vi "MainVI_IRVision.vi"() -> ()   [LabVIEW 2013]
uses:
  StateEnum.ctl
  StateImageQueue.ctl
  Parameter.ctl
  <vilib>/picture/picture.llb/imagedata.ctl
  <vilib>/Analysis/baseanly.llb/Mean (DBL).vi
  <vilib>/Analysis/NI_AALBase.lvlib
panel:
  out "error out 2":errorcluster caption="error out"
  out "error out":errorcluster
  in  "UPDATE - Button":bool
  out "IRImage Width":i32
  out "IRImage Height":i32
  in  "Camera":u32(ring) items=["t890-2(2131919)"=2131919]
  out "MEASUREMENT RANGES":u32
  out "Min. Value":sgl format="%#_2f"
  out "Max. Value":sgl format="%#_2f"
  out "Mean":dbl caption="Mittelwert" format="%0.2f"
  in  "PaletteType":u8(ring) items=["Iron", "Rainbow", "BlueRed", "Testo", "Sepia", "Dewpoint", "RainbowHC"]
  out "IsStreaming":bool
  out "CONNECTED":bool caption="l"
  in  "STOP - Button":bool
  in  "SAVE - Button":bool
  in  "CONNECT - Button":bool
  in  "STREAM - Button":bool
  in  "EXIT - Button":bool
  in  "ATMOSPHERECORRECTION":bool
  in  "AMBIENTTEMPERATURE":sgl
  in  "HUMIDITY":sgl
  in  "MEASUREMENT RANGE":u32
  in  "REFLECTEDTEMPERATURE":sgl
  in  "EMISSIVITY":sgl=0.3 format="%.2f"
  out "IR Image":picture
  # "Testo 885, 890"
  # "CONNECTION"
  # "STREAM"
  # "PARAMETER"
  # "IR IMAGE"
  # "Measurement Ranges"
  # "Palette Type"
  # "Measurement Range"
  # "Height"
  # "Humidity"
  # "Width"
  # "Ambient Temperature"
  # "Min. Value"
  # "Emissivity"
  # "Max. Value"
  # "Reflected Temperature"
  # "Mean Value"
  # "Atmosphere Correction"
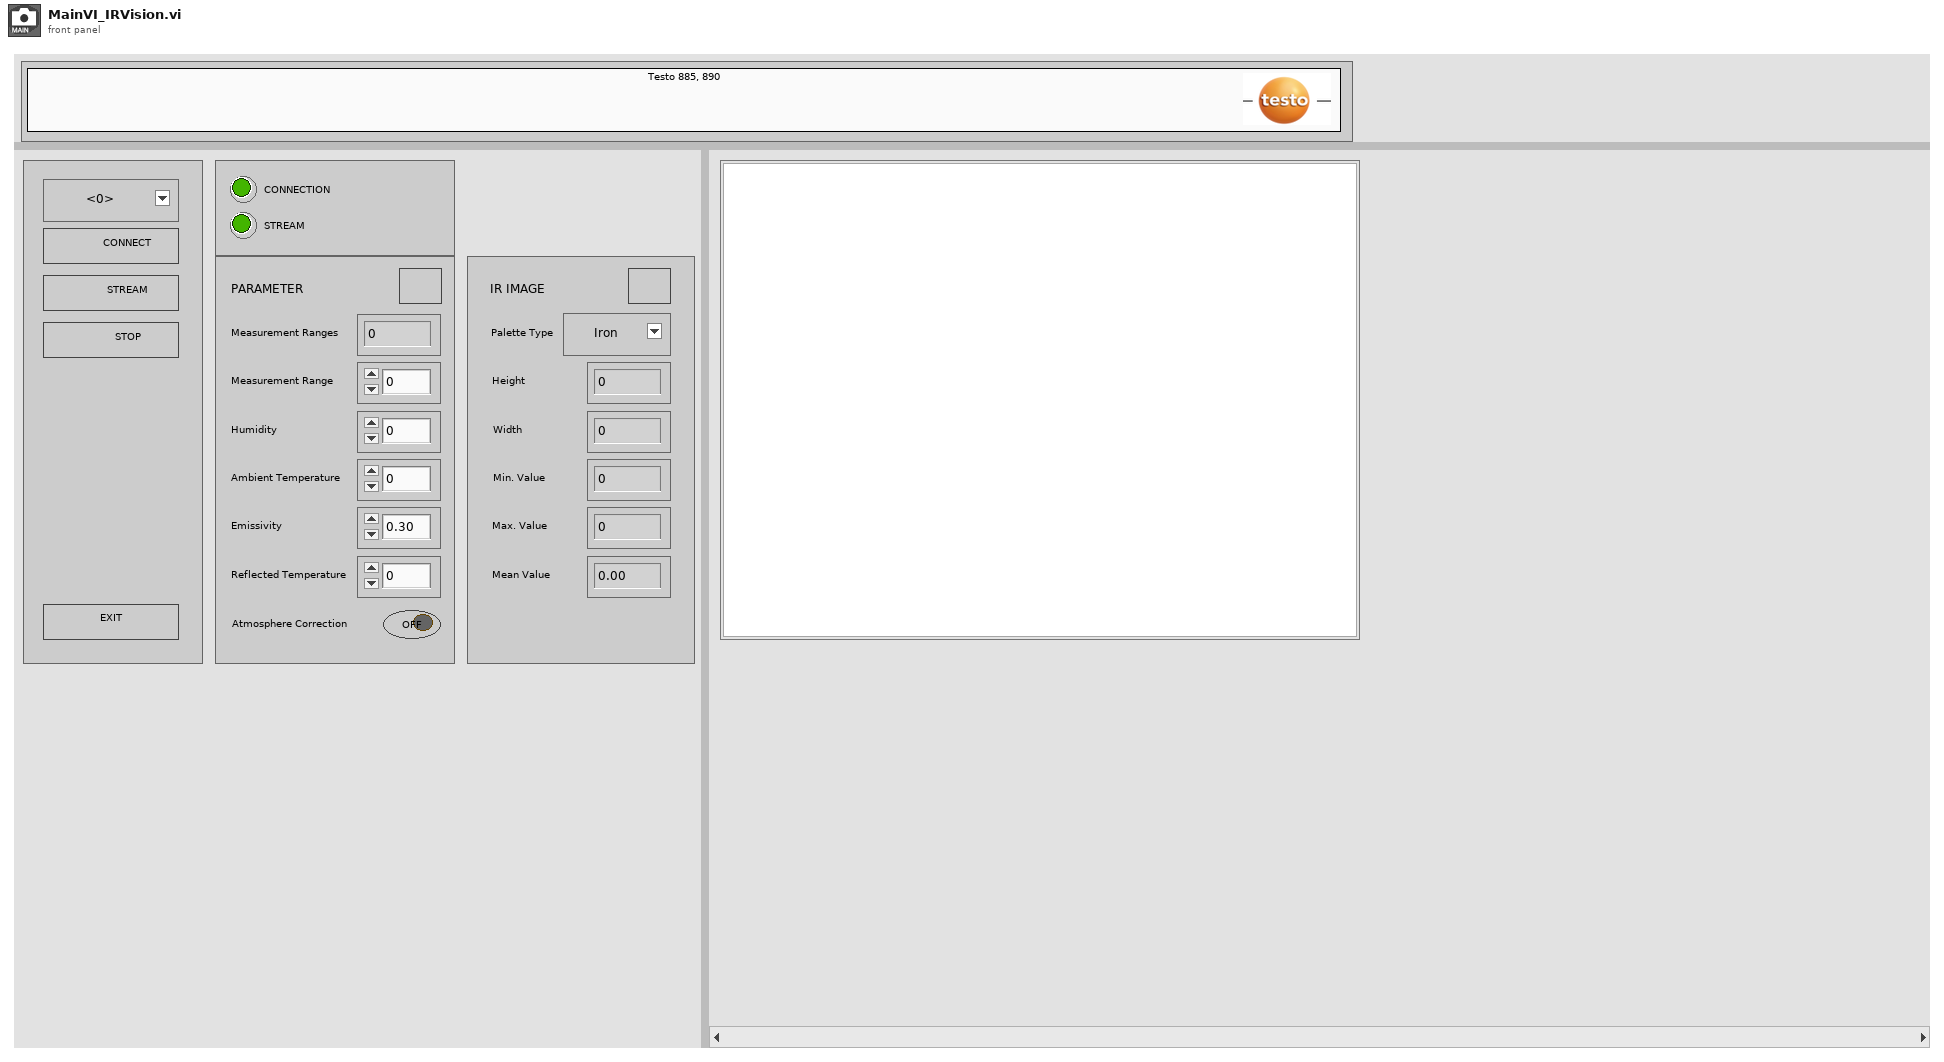
[diagram p1: front panel]
types:
  T1 = typedef "StateImageQueue.ctl" = enum16{"INITIALIZE", "GET IMAGE", "IDLE", "GET STREAM", "EXIT", ""}
  T2 = typedef "StateEnum.ctl" = enum16{"INITIALIZE", "CONNECT", "STREAM", "STOPSTREAM", "GETIMAGES", "SETPARAMTER", "GETPARAMETER", "SAVEIMAGE", "EXIT"}
  T3 = cluster{"IR QUEUE":refnum<queue>, "VIS QUEUE":refnum<queue>}
  T4 = typedef "Parameter.ctl" = enum16{"EMISSIVITY", "ATMOSPHERECORRECTION", "HUMIDITY", "REFLECTEDTEMPERATURE", "AMBIENTTEMPERATURE", "MEASUREMENTRANGE"}
  T5 = typedef "imagedata.ctl" = cluster{"image type":i32, "image depth":i32, "image":u8[], "mask":u8[], "colors":u32[], "Rectangle":cluster{"left":i16, "top":i16, "right":i16, "bottom":i16}}
  T6 = cluster{"left":i16, "top":i16, "right":i16, "bottom":i16}
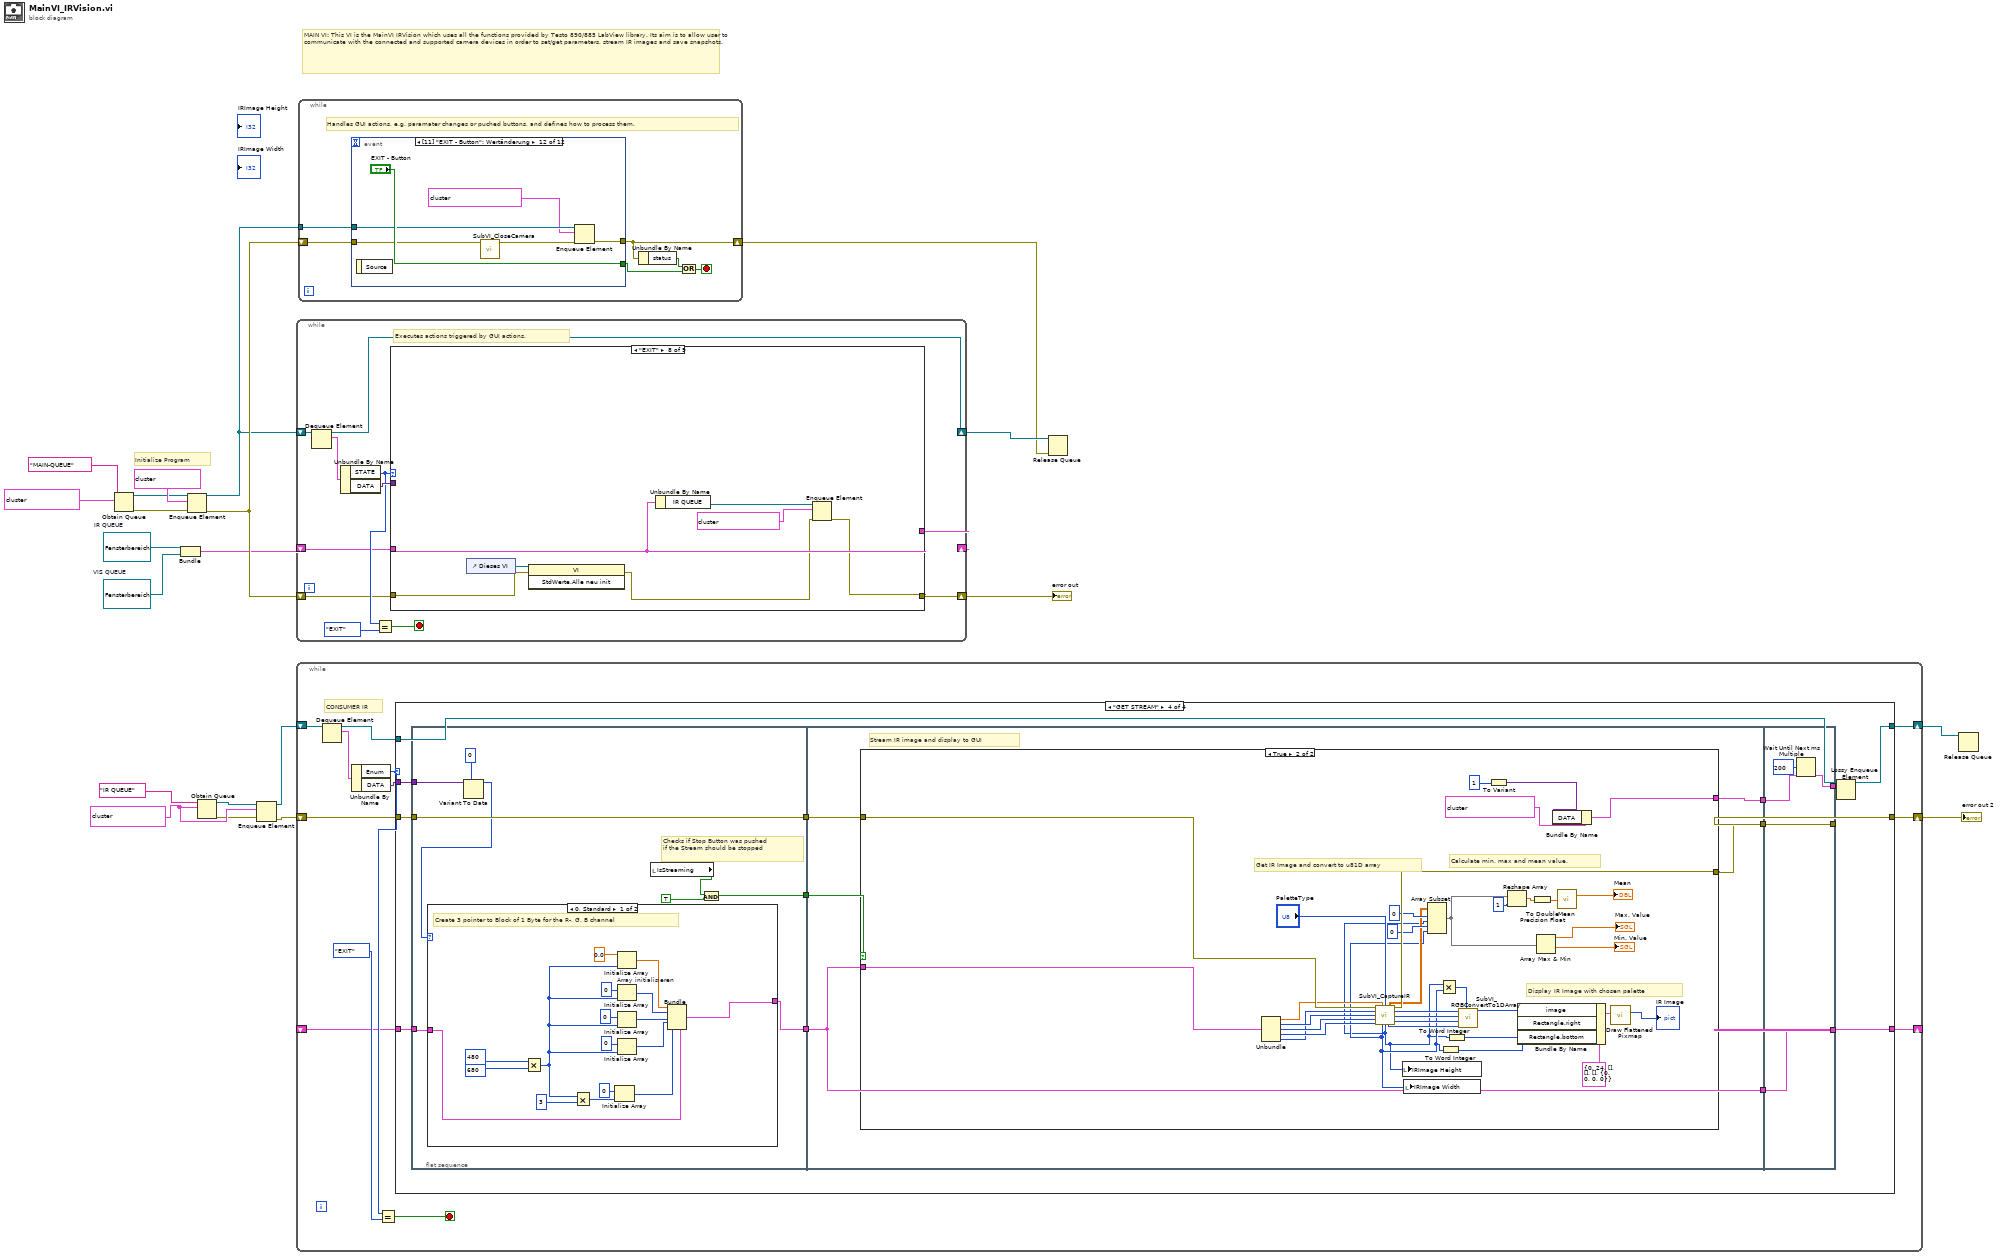
[diagram p0: block diagram]
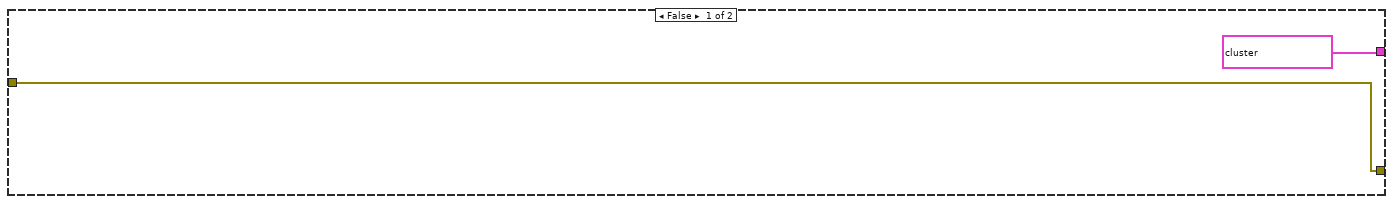
[diagram p6: hidden frame]
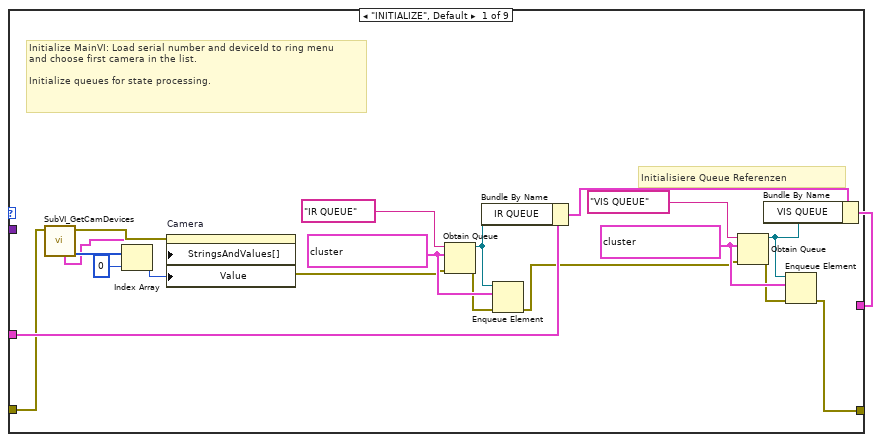
[diagram p7: hidden frame]
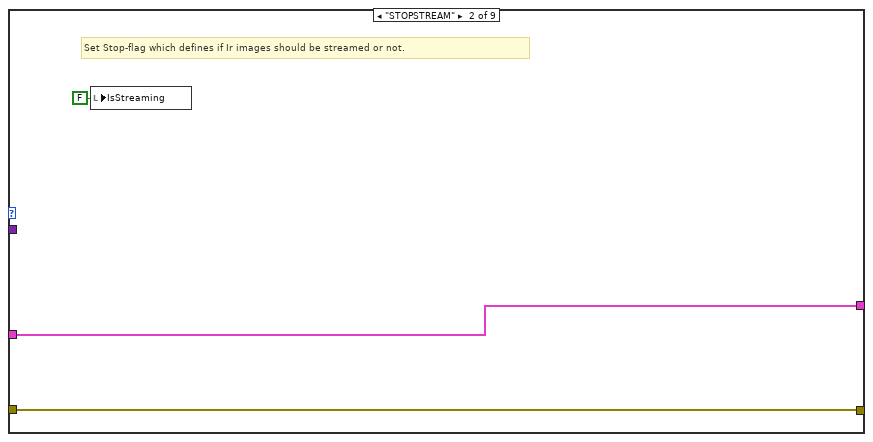
[diagram p8: hidden frame]
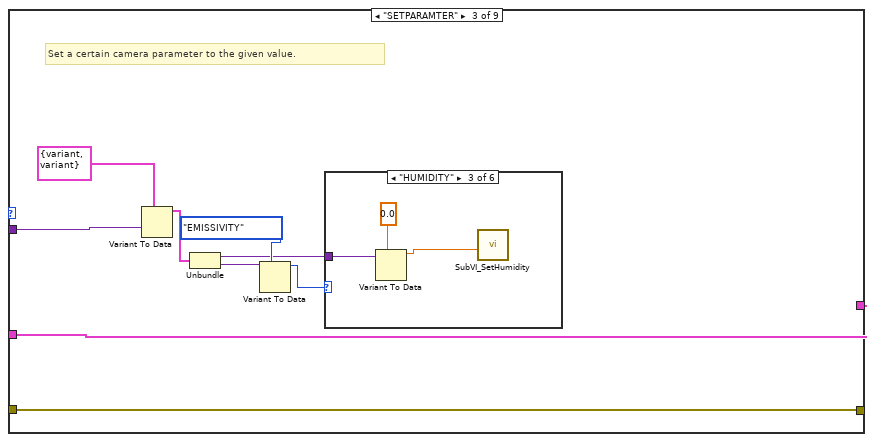
[diagram p9: hidden frame]
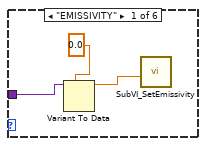
[diagram p10: hidden frame]
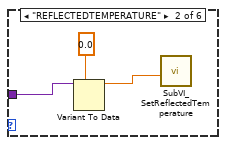
[diagram p11: hidden frame]
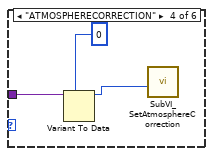
[diagram p12: hidden frame]
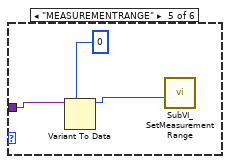
[diagram p13: hidden frame]
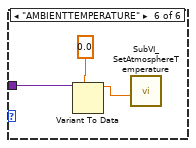
[diagram p14: hidden frame]
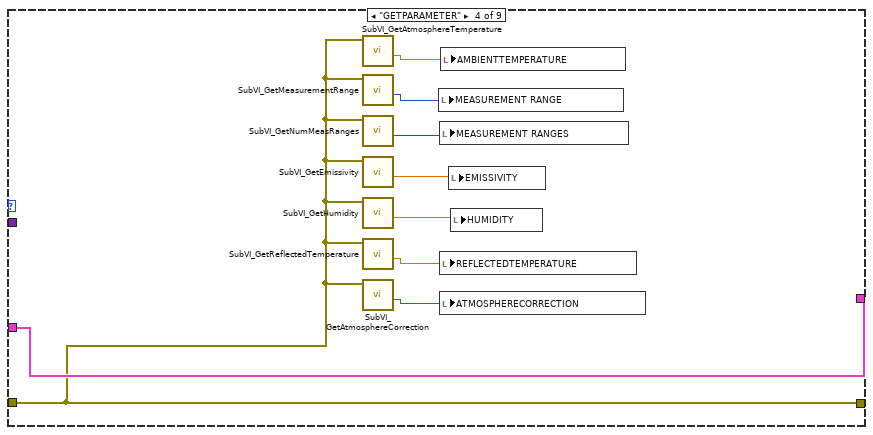
[diagram p15: hidden frame]
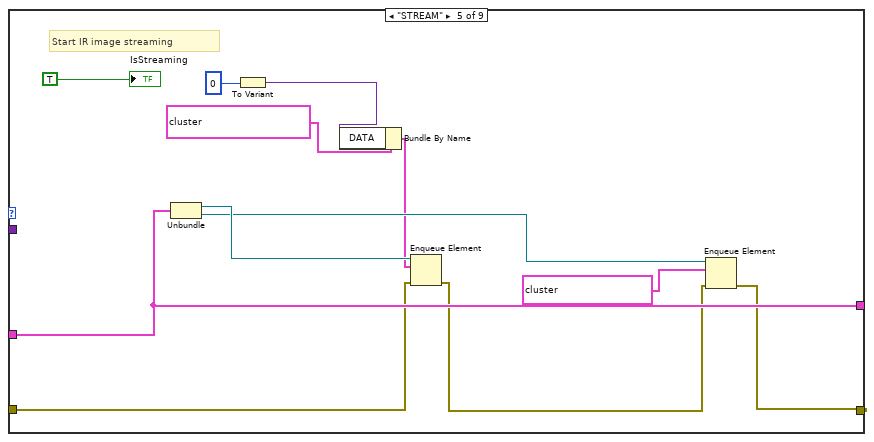
[diagram p16: hidden frame]
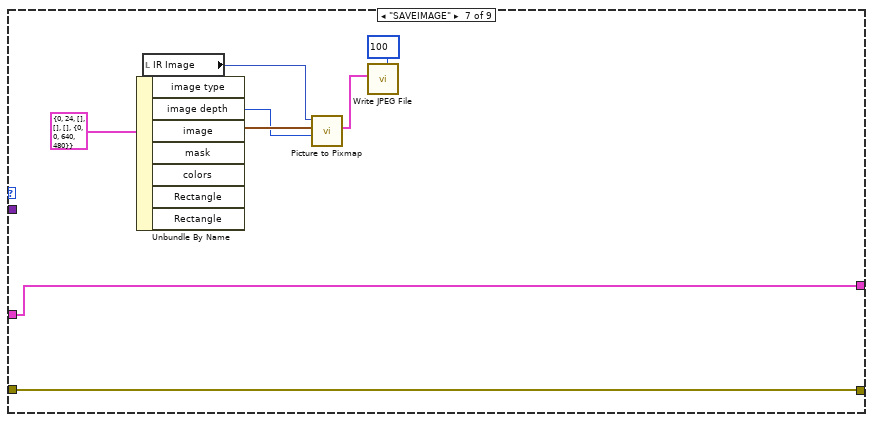
[diagram p18: hidden frame]
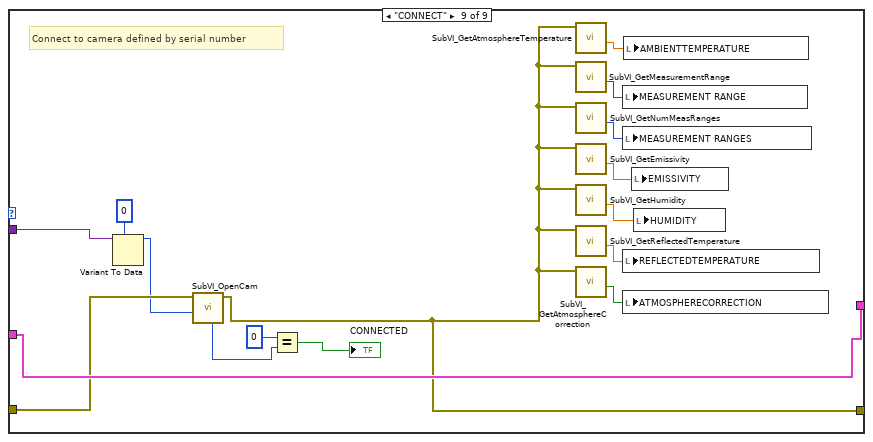
[diagram p19: hidden frame]
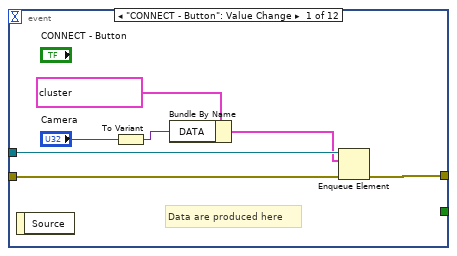
[diagram p20: hidden frame]
diagram:
  w3 = refnum<queue> refnum  # VIS QUEUE
  w7 = refnum<queue> refnum  # IR QUEUE
  w13 = cluster{"DATA":variant, "Enum":T1} {"DATA"=variant, "Enum"=enum."INITIALIZE"}
  # "Initialize Program"
  # "MAIN VI: This VI is the MainVI IRVision which uses all the functions provided by Testo 890/885 LabView library. Its aim is to allow user to communicate with the connected and supported camera devices in order to set/get parameters, stream IR images and save snapshots."
  n1 = Obtain Queue(name (unnamed)="MAIN-QUEUE" ("Name (unbenannt)"), element data type=cluster{"DATA":variant, "STATE":T2} {"DATA"=variant, "STATE"=enum."INITIALIZE"}) -> (queue out=w18:refnum<queue>, error out=w17:errorcluster)  [unwired: 3 in, 1 out]
  n2 = Bundle("IR QUEUE"=w7, "VIS QUEUE"=w3) -> (w6:T3)  [unwired: 1 in]
  n3 = Enqueue Element(queue=w18, element=cluster{"DATA":variant, "STATE":T2} {"DATA"=variant, "STATE"=enum."INITIALIZE"} ("Element"), error in (no error)=w17) -> (queue out=w11:refnum<queue>, error out=w16:errorcluster)  [unwired: 1 in, 1 out]
  n4 = Obtain Queue(name (unnamed)="IR QUEUE" ("Name (unbenannt)"), element data type=w13) -> (queue out=w14:refnum<queue>, error out=w12:errorcluster)  [unwired: 3 in, 1 out]
  n5 = Enqueue Element(queue=w14, element=w13, error in (no error)=w12) -> (queue out=w5:refnum<queue>, error out=w4:errorcluster)  [unwired: 1 in, 1 out]
  n6 = while {
    shift-right: [w24] -> w1
    shift-left: w16 -> [w27]
    shift-right: [w22] -> w10
    shift-left: w11 -> [w32]
    shift-right: [w25] -> _
    shift-left: w6 -> [w26]
    stop <- w23 stop-if-true
    # "Executes actions triggered by GUI actions."
    n7 = Dequeue Element(queue=w32) -> (queue out=w22:refnum<queue>, element=w31:cluster{"DATA":variant, "STATE":T2})  [unwired: 2 in, 2 out]
    n8 = Unbundle By Name(w31) -> ("STATE"=w29:T2, "DATA"=w30:variant)
    n9 = Equal?(x=w29, y=StateEnum."EXIT") -> (x = y?=w23:bool)
    n10 = case shown="\"EXIT\"" w29 {
      tunnel: w30 -> [_ _ w64 _ _ _ _ _ w135]
      tunnel: w27 -> [w34 w54 w56 w90 w101 w104 w106 w116 w133]
      tunnel: [w38 w54 w56 w90 w96 w104 w106 w114 w132] -> w24
      tunnel: w26 -> [w47 w55 w63 w91 w103 w105 w107 w118 w134]
      tunnel: [w35 w55 w63 w91 w103 w105 w107 w118 w134] -> w25
      frame "INITIALIZE", Default {
        w41 = cluster{"DATA":variant, "Enum":T1} {"DATA"=variant, "Enum"=enum."INITIALIZE"}
        w46 = cluster{"DATA":variant, "Enum":T1} {"DATA"=variant, "Enum"=enum."INITIALIZE"}
        # "Initialisiere Queue Referenzen"
        # "Initialize MainVI: Load serial number and deviceId to ring menu\nand choose first camera in the list.\n\nInitialize queues for state processing."
        n11 = call "SubVI_GetCamDevices.vi"("ErrorIn"=w34) -> ("au32CameraSerials"=w51:u32[], "ErrorOut"=w49:errorcluster, "strCameraDeviceType"=w33:cluster{string, "Output":u32}[])  [unwired: 6 in, 2 out]
        n12 = Index Array(array=w51, index=0 ("Index")) -> (element=w52:u32)
        n13 = property on="Camera" class="Ring (strikt)"(error in=w49, "StringsAndValues[]"=w33, "Value"=w52) -> (error out=w43:errorcluster)  [unwired: 1 in, 1 out]
        n14 = Obtain Queue ("Queue anfordern")(name (unnamed)="IR QUEUE" ("Name (unbenannt)"), element data type=w46, error in (no error)=w43) -> (queue out=w45:refnum<queue>, error out=w44:errorcluster)  [unwired: 2 in, 1 out]
        n15 = Bundle By Name(cluster=w47, "IR QUEUE"=w45) -> (w36:T3)
        n16 = Enqueue Element(queue=w45, element=w46, error in (no error)=w44) -> (error out=w39:errorcluster)  [unwired: 1 in, 2 out]
        n17 = Obtain Queue ("Queue anfordern")(name (unnamed)="VIS QUEUE" ("Name (unbenannt)"), element data type=w41, error in (no error)=w39) -> (queue out=w37:refnum<queue>, error out=w40:errorcluster)  [unwired: 2 in, 1 out]
        n18 = Bundle By Name(cluster=w36, "VIS QUEUE"=w37) -> (w35:T3)
        n19 = Enqueue Element(queue=w37, element=w41, error in (no error)=w40) -> (error out=w38:errorcluster)  [unwired: 1 in, 2 out]
      }
      frame "STOPSTREAM" {
        # "Set Stop-flag which defines if Ir images should be streamed or not."
        n20 = local write "IsStreaming"(FALSE) -> ()
      }
      frame "SETPARAMTER" {
        # "Set a certain camera parameter to the given value."
        n21 = Variant To Data(type=cluster{variant, variant} {variant, variant}, Variant=w64) -> (data=w61:cluster{variant, variant})  [unwired: 1 in, 1 out]
        n22 = Unbundle(w61) -> (w57:variant, w58:variant)
        n23 = Variant To Data(type=Parameter."EMISSIVITY" ("Enum"), Variant=w58) -> (data=w59:T4)  [unwired: 1 in, 1 out]
        n24 = case shown="\"HUMIDITY\"" w59 {
          tunnel: w57 -> [w67 w69 w72 w76 w78 w81]
          frame "EMISSIVITY" {
            n25 = Variant To Data(type=sgl 0.0, Variant=w67) -> (data=w65:sgl)  [unwired: 1 in, 1 out]
            n26 = call "SubVI_SetEmissivity.vi"("fEmissivity"=w65) -> ()  [unwired: 9 in, 2 out]
          }
          frame "REFLECTEDTEMPERATURE" {
            n27 = Variant To Data(type=sgl 0.0, Variant=w69) -> (data=w68:sgl)  [unwired: 1 in, 1 out]
            n28 = call "SubVI_SetReflectedTemperature.vi"("fReflectedTemp"=w68) -> ()  [unwired: 9 in, 2 out]
          }
          frame "HUMIDITY" {
            n29 = Variant To Data(type=sgl 0.0, Variant=w72) -> (data=w71:sgl)  [unwired: 1 in, 1 out]
            n30 = call "SubVI_SetHumidity.vi"("fHumidity"=w71) -> ()  [unwired: 9 in, 2 out]
          }
          frame "ATMOSPHERECORRECTION" {
            n31 = Variant To Data(type=u8 0, Variant=w76) -> (data=w74:u8)  [unwired: 1 in, 1 out]
            n32 = call "SubVI_SetAtmosphereCorrection.vi"("u8AtmosCorrEnable"=w74) -> ()  [unwired: 9 in, 2 out]
          }
          frame "MEASUREMENTRANGE" {
            n33 = Variant To Data(type=u32 0, Variant=w78) -> (data=w77:u32)  [unwired: 1 in, 1 out]
            n34 = call "SubVI_SetMeasurementRange.vi"("u32MeasurementRange"=w77) -> ()  [unwired: 9 in, 2 out]
          }
          frame "AMBIENTTEMPERATURE" {
            n35 = Variant To Data(type=sgl 0.0, Variant=w81) -> (data=w80:sgl)  [unwired: 1 in, 1 out]
            n36 = call "SubVI_SetAtmosphereTemperature.vi"("fAtmosTemp"=w80) -> ()  [unwired: 9 in, 2 out]
          }
        }
      }
      frame "GETPARAMETER" {
        n37 = call "SubVI_GetAtmosphereTemperature.vi"("ErrorIn"=w90) -> ("fAtmosTemp"=w89:sgl)  [unwired: 8 in, 2 out]
        n38 = call "SubVI_GetMeasurementRange.vi"("ErrorIn"=w90) -> ("u32MeasRangeIndex"=w88:u32)  [unwired: 8 in, 2 out]
        n39 = call "SubVI_GetNumMeasRanges.vi"("ErrorIn"=w90) -> ("u32NumMeasRanges"=w87:u32)  [unwired: 8 in, 2 out]
        n40 = call "SubVI_GetEmissivity.vi"("ErrorIn"=w90) -> ("fEmissivity"=w86:sgl)  [unwired: 8 in, 2 out]
        n41 = call "SubVI_GetHumidity.vi"("ErrorIn"=w90) -> ("fHumidity"=w85:sgl)  [unwired: 8 in, 2 out]
        n42 = call "SubVI_GetReflectedTemperature.vi"("ErrorIn"=w90) -> ("fReflectedTemp"=w84:sgl)  [unwired: 8 in, 2 out]
        n43 = call "SubVI_GetAtmosphereCorrection.vi"("ErrorIn"=w90) -> ("bAtmosCorrEnable"=w83:bool)  [unwired: 8 in, 2 out]
        n44 = local write "MEASUREMENT RANGE"(w88) -> ()
        n45 = local write "MEASUREMENT RANGES"(w87) -> ()
        n46 = local write "REFLECTEDTEMPERATURE"(w84) -> ()
        n47 = local write "ATMOSPHERECORRECTION"(w83) -> ()
        n48 = local write "AMBIENTTEMPERATURE"(w89) -> ()
        n49 = local write "EMISSIVITY"(w86) -> ()
        n50 = local write "HUMIDITY"(w85) -> ()
      }
      frame "STREAM" {
        # "Start IR image streaming"
        n51 = Unbundle(w103) -> ("IR QUEUE"=w102:refnum<queue>, "VIS QUEUE"=w98:refnum<queue>)
        n52 = To Variant(anything=u8 0) -> (Variant=w95:variant)
        n53 = Bundle By Name(cluster=cluster{"DATA":variant, "Enum":T1} {"DATA"=variant, "Enum"=enum."GET STREAM"}, "DATA"=w95) -> (w92:cluster{"DATA":variant, "Enum":T1})
        n54 = Enqueue Element(queue=w102, element=w92, error in (no error)=w101) -> (error out=w97:errorcluster)  [unwired: 1 in, 2 out]
        n55 = Enqueue Element(queue=w98, element=cluster{"DATA":variant, "Enum":T1} {"DATA"=variant, "Enum"=enum."GET STREAM"}, error in (no error)=w97) -> (error out=w96:errorcluster)  [unwired: 1 in, 2 out]
        "IsStreaming" <- TRUE
      }
      frame "GETIMAGES" {
      }
      frame "SAVEIMAGE" {
        n56 = Unbundle By Name(T5 {"image type"=0, "image depth"=24, "image"=[], "mask"=[], "colors"=[], "Rectangle"={"left"=0, "top"=0, "right"=640, "bottom"=480}} ("image data")) -> ("image depth"=w110:i32, "Rectangle"=w112:T6)  [unwired: 5 out]
        n57 = local read "IR Image"() -> (w111:picture)
        n58 = call <vilib>:"Picture to Pixmap.vi"("depth"=w110, "rect"=w112, "picture"=w111) -> ("image data"=w109:T5)  [unwired: 7 in, 1 out]
        n59 = call <vilib>:"Write JPEG File.vi"("quality (80)"=100, "image data"=w109) -> ()  [unwired: 8 in, 2 out]
      }
      frame "EXIT" {
        n60 = control-ref of="Dieses VI"() -> (w117:refnum<vi>)
        n61 = invoke class="VI" method="StdWerte.Alle neu init"(reference=w117, error in=w116) -> (error out=w115:errorcluster)  [unwired: 1 in, 2 out]
        n62 = Unbundle By Name(w118) -> ("IR QUEUE"=w119:refnum<queue>)
        n63 = Enqueue Element(queue=w119, element=cluster{"DATA":variant, "Enum":T1} {"DATA"=variant, "Enum"=enum."EXIT"}, error in (no error)=w115) -> (error out=w114:errorcluster)  [unwired: 1 in, 2 out]
      }
      frame "CONNECT" {
        # "Connect to camera defined by serial number"
        n64 = Variant To Data(type=u32 0 ("Typ"), Variant=w135) -> (data=w131:u32)  [unwired: 1 in, 1 out]
        n65 = call "SubVI_OpenCam.vi"("u32SerialNumber"=w131, "ErrorIn"=w133) -> ("ErrorOut"=w132:errorcluster, "u8Status"=w123:u8)  [unwired: 8 in]
        n66 = Equal?(x=u8 0, y=w123) -> (x = y?=→"CONNECTED":bool)
        n67 = call "SubVI_GetAtmosphereTemperature.vi"("ErrorIn"=w132) -> ("fAtmosTemp"=w124:sgl)  [unwired: 8 in, 2 out]
        n68 = call "SubVI_GetMeasurementRange.vi"("ErrorIn"=w132) -> ("u32MeasRangeIndex"=w125:u32)  [unwired: 8 in, 2 out]
        n69 = call "SubVI_GetNumMeasRanges.vi"("ErrorIn"=w132) -> ("u32NumMeasRanges"=w126:u32)  [unwired: 8 in, 2 out]
        n70 = call "SubVI_GetEmissivity.vi"("ErrorIn"=w132) -> ("fEmissivity"=w127:sgl)  [unwired: 8 in, 2 out]
        n71 = call "SubVI_GetHumidity.vi"("ErrorIn"=w132) -> ("fHumidity"=w128:sgl)  [unwired: 8 in, 2 out]
        n72 = call "SubVI_GetReflectedTemperature.vi"("ErrorIn"=w132) -> ("fReflectedTemp"=w129:sgl)  [unwired: 8 in, 2 out]
        n73 = call "SubVI_GetAtmosphereCorrection.vi"("ErrorIn"=w132) -> ("bAtmosCorrEnable"=w130:bool)  [unwired: 8 in, 2 out]
        n74 = local write "MEASUREMENT RANGE"(w125) -> ()
        n75 = local write "MEASUREMENT RANGES"(w126) -> ()
        n76 = local write "REFLECTEDTEMPERATURE"(w129) -> ()
        n77 = local write "ATMOSPHERECORRECTION"(w130) -> ()
        n78 = local write "AMBIENTTEMPERATURE"(w124) -> ()
        n79 = local write "EMISSIVITY"(w127) -> ()
        n80 = local write "HUMIDITY"(w128) -> ()
      }
    }
  }
  "error out" <- w1
  n81 = while {
    shift-right: [w137] -> w8
    shift-left: w5 -> [w144]
    shift-right: [w142] -> w2
    shift-left: w4 -> [w141]
    shift-right: [w139] -> _
    shift-left: _ -> [w140]
    stop <- w146 stop-if-true
    # "CONSUMER IR"
    n82 = Dequeue Element(queue=w144) -> (queue out=w138:refnum<queue>, element=w148:cluster{"DATA":variant, "Enum":T1})  [unwired: 2 in, 2 out]
    n83 = Unbundle By Name(w148) -> ("Enum"=w145:T1, "DATA"=w147:variant)
    n84 = Equal?(x=w145, y=StateImageQueue."EXIT" ("Enum 2")) -> (x = y?=w146:bool)
    n85 = case shown="\"GET STREAM\"" w145 {
      tunnel: w147 -> [_ _ _ w158]
      tunnel: [w151 w154 w157 w168] -> w142
      tunnel: w141 -> [w151 w154 w157 w170]
      tunnel: w140 -> [w150 w152 w156 w167]
      tunnel: [w150 w152 w156 w166] -> w139
      tunnel: w138 -> [w149 w153 w155 w162]
      tunnel: [w149 w153 w155 w163] -> w137
      frame "INITIALIZE", Default {
        # "Initialize ring menu with serial numbers\nand choose first camera in the list"
      }
      frame "IDLE" {
      }
      frame "GET IMAGE" {
      }
      frame "GET STREAM" {
        n86 = flat-sequence {
          tunnel: w167 -> [w172]
          tunnel: w170 -> [w180]
          tunnel: [w180] -> w161
          tunnel: [w173] -> w160
          tunnel: [w177] -> w159
          tunnel: w158 -> [w175]
          tunnel: [w201] -> w171
          tunnel: [w202] -> w169
          tunnel: [w200] -> w165
          tunnel: w161 -> [w203]
          tunnel: w160 -> [w200]
          tunnel: w159 -> [w199]
          tunnel: w171 -> [w241]
          tunnel: w169 -> [w243]
          tunnel: [w243] -> w168
          tunnel: [w244] -> w166
          tunnel: w165 -> [w244]
          tunnel: [w241] -> w164
          frame #0 {
            # "Checks if Stop Button was pushed\nif the Stream should be stopped"
            n87 = Variant To Data(type=u8 0 ("Typ"), Variant=w175) -> (data=w174:u8)  [unwired: 1 in, 1 out]
            n88 = case shown="0, Standard" w174 {
              tunnel: [w187 w198] -> w173
              tunnel: w172 -> [w186 w198]
              frame 0, Default {
                # "Create 3 pointer to Block of 1 Byte for the R-, G, B channel"
                n89 = Multiply(x=480, y=680 ("x")) -> (x*y=w182:i32)
                n90 = Multiply(x=w182, y=3) -> (x*y=w192:i32)
                n91 = Initialize Array(u8 0 ("Element"), w192) -> (w188:u8[])
                n92 = Initialize Array(sgl 0.0 ("Element"), w182) -> (w181:sgl[])
                n93 = Initialize Array "Array initialisieren"(u8 0 ("Element"), w182) -> (w191:u8[])
                n94 = Initialize Array(u8 0 ("Element"), w182) -> (w190:u8[])
                n95 = Initialize Array(u8 0 ("Element"), w182) -> (w189:u8[])
                n96 = Bundle(cluster=w186, w181, w191, w190, w189, w188) -> (w187:cluster{sgl[], u8[], u8[], u8[], u8[]})
              }
              frame 1 {
              }
            }
            n97 = local read "IsStreaming"() -> (w179:bool)
            n98 = And(x=w179, y=TRUE) -> (x .and. y?=w177:bool)
          }
          frame #1 {
            # "Stream IR image and display to GUI"
            n99 = case shown="True" w199 {
              tunnel: w203 -> [w204 w240]
              tunnel: [w204 w239] -> w202
              tunnel: [cluster{"DATA":variant, "Enum":T1} {"DATA"=variant, "Enum"=enum."IDLE"} w216] -> w201
              tunnel: w200 -> [_ w238]
              frame False {
              }
              frame True {
                # "Get IR Image and convert to u81D array"
                # "Calculate min, max and mean value."
                # "Display IR Image with chosen palette"
                n100 = Unbundle(w238) -> (w233:sgl[], w232:u8[], w231:u8[], w230:u8[], w229:u8[])
                n101 = call "SubVI_CaptureIR.vi"("ErrorIn"=w240, "af1DTempMat"=w233, "u8PaletteType"="PaletteType", "au8Channel-B"=w232, "au8Channel-G"=w231, "au8Channel-R"=w230) -> ("af2DTempMat"=w209:sgl[][], "ErrorOut"=w239:errorcluster, "au8Channel-B"=w235:u8[], "au8Channel-G"=w236:u8[], "i32Width"=w207:i32, "i32Height"=w206:i32, "au8Channel-R"=w237:u8[])  [unwired: 2 in, 1 out]
                n102 = local write "IRImage Height"(w206) -> ()
                n103 = local write "IRImage Width"(w207) -> ()
                n104 = Array Subset(array=w209, index (row)=0 ("Index"), length (row)=w206, index (col)=0 ("Index"), length (col)=w207) -> (w208:sgl[][])
                n105 = Multiply(x=w206, y=w207) -> (x*y=w234:i32)
                n106 = To Word Integer(number=w207) -> (16bit integer=w213:i16)
                n107 = To Word Integer(number=w206) -> (16bit integer=w212:i16)
                n108 = call "SubVI_RGBConvertTo1DArray.vi"("i32PixelAmount"=w234, "au8Channel-R"=w237, "au8Channel-G"=w236, "au8Channel-B"=w235, "au8SerializedImage[in]"=w229) -> ("au8SerializedImage[out]"=w226:u8[])  [unwired: 6 in]
                n109 = To Variant(anything=u8 1) -> (Variant=w218:variant)
                n110 = Reshape Array(w208, 1 ("Dimension")) -> (w222:sgl[])
                n111 = Bundle By Name(cluster=T5 {"image type"=0, "image depth"=24, "image"=[], "mask"=[], "colors"=[], "Rectangle"={"left"=0, "top"=0, "right"=0, "bottom"=0}} ("image data"), "image"=w226, "Rectangle.right"=w213, "Rectangle.bottom"=w212) -> (w224:T5)
                n112 = To Double Precision Float(number=w222) -> (double precision float=w223:dbl[])
                n113 = Array Max & Min(array=w208) -> (max value=→"Max. Value":sgl, min value=→"Min. Value":sgl)  [unwired: 2 out]
                n114 = Bundle By Name(cluster=cluster{"DATA":variant, "Enum":T1} {"DATA"=variant, "Enum"=enum."GET STREAM"}, "DATA"=w218) -> (w216:cluster{"DATA":variant, "Enum":T1})
                n115 = call-poly <vilib>:"Mean.vi"("X"=w223) -> ("mean"=→"Mean":dbl)  [unwired: 1 out]
                n116 = call <vilib>:"Draw Flattened Pixmap.vi"("image data"=w224) -> ("new picture"=→"IR Image":picture)  [unwired: 8 in]
              }
            }
          }
          frame #2 {
            n117 = Wait Until Next ms Multiple(millisecond multiple=u32 200 ("ms")) -> ()  [unwired: 1 out]
          }
        }
        n118 = Lossy Enqueue Element(queue=w162, element=w164) -> (queue out=w163:refnum<queue>)  [unwired: 1 in, 3 out]
      }
    }
  }
  "error out 2" <- w2
  n119 = while {
    shift-right: [w245] -> w9
    shift-left: w16 -> [w249]
    tunnel: w11 -> [w250]
    stop <- w248 stop-if-true
    # "Handles GUI actions, e.g. paramater changes or puched buttons, and defines how to process them."
    n120 = event shown="[11] \"EXIT - Button\": Wertänderung" {
      selector: _ -> [_ _ _ _ _ _ _ _ _ _ _ _]
      dyn-events: _ -> [_ _ _ _ _ _ _ _ _ _ _ _]
      timeout: _ -> [_ _ _ _ _ _ _ _ _ _ _ _]
      tunnel: w250 -> [w257 w260 w264 w266 w273 w287 w296 w304 w310 w312 w323 w334]
      tunnel: w249 -> [w256 w261 w263 w267 w272 w286 w295 w303 w309 w313 w322 w331]
      tunnel: [_ _ _ _ _ _ _ _ _ _ _ "EXIT - Button"] -> w246
      tunnel: [w255 w259 w262 w268 w271 w285 w294 w300 w308 w314 w321 w333] -> w245
      event "CONNECT - Button": Value Change {
        # "Data are produced here"
        n121 = event-data() -> ()  [unwired: 1 in, 1 out]
        n122 = To Variant(anything="Camera") -> (Variant=w252:variant)
        n123 = Bundle By Name(cluster=cluster{"DATA":variant, "STATE":T2} {"DATA"=variant, "STATE"=enum."CONNECT"} ("Element"), "DATA"=w252) -> (w251:cluster{"DATA":variant, "STATE":T2})
        n124 = Enqueue Element(queue=w257, element=w251, error in (no error)=w256) -> (error out=w255:errorcluster)  [unwired: 1 in, 2 out]
      }
      event "STREAM - Button": Value Change {
        n125 = event-data() -> ()  [unwired: 1 in, 1 out]
        n126 = Enqueue Element(queue=w260, element=cluster{"DATA":variant, "STATE":T2} {"DATA"=variant, "STATE"=enum."STREAM"} ("Element"), error in (no error)=w261) -> (error out=w259:errorcluster)  [unwired: 1 in, 2 out]
      }
      event "STOP - Button": Value Change {
        n127 = event-data() -> ()  [unwired: 1 in, 1 out]
        n128 = Enqueue Element(queue=w264, element=cluster{"DATA":variant, "STATE":T2} {"DATA"=variant, "STATE"=enum."STOPSTREAM"} ("Element"), error in (no error)=w263) -> (error out=w262:errorcluster)  [unwired: 1 in, 2 out]
      }
      event "UPDATE - Button": Value Change {
        n129 = event-data() -> ()  [unwired: 1 in, 1 out]
        n130 = Enqueue Element(queue=w266, element=cluster{"DATA":variant, "STATE":T2} {"DATA"=variant, "STATE"=enum."GETPARAMETER"} ("Element"), error in (no error)=w267) -> (error out=w268:errorcluster)  [unwired: 1 in, 2 out]
      }
      event "MEASUREMENT RANGE": Value Change {
        n131 = event-data() -> ()  [unwired: 1 in, 1 out]
        n132 = Bundle("MEASUREMENT RANGE"="MEASUREMENT RANGE", Parameter."MEASUREMENTRANGE") -> (w275:cluster{"MEASUREMENT RANGE ":u32, T4})  [unwired: 1 in]
        n133 = To Variant(anything=w275) -> (Variant=w274:variant)
        n134 = Bundle By Name(cluster=cluster{"DATA":variant, "STATE":T2} {"DATA"=variant, "STATE"=enum."SETPARAMTER"} ("Element"), "DATA"=w274) -> (w278:cluster{"DATA":variant, "STATE":T2})
        n135 = Enqueue Element(queue=w273, element=w278, error in (no error)=w272) -> (error out=w271:errorcluster)  [unwired: 1 in, 2 out]
      }
      event "ATMOSPHERECORRECTION": Value Change {
        n136 = event-data() -> ()  [unwired: 1 in, 1 out]
        n137 = Boolean To (0,1)(Boolean="ATMOSPHERECORRECTION") -> (0, 1=w279:i16)
        n138 = To Unsigned Byte Integer(number=w279) -> (unsigned 8bit integer=w281:u8)
        n139 = Bundle(w281, Parameter."ATMOSPHERECORRECTION") -> (w283:cluster{u8, T4})  [unwired: 1 in]
        n140 = To Variant(anything=w283) -> (Variant=w282:variant)
        n141 = Bundle By Name(cluster=cluster{"DATA":variant, "STATE":T2} {"DATA"=variant, "STATE"=enum."SETPARAMTER"} ("Element"), "DATA"=w282) -> (w288:cluster{"DATA":variant, "STATE":T2})
        n142 = Enqueue Element(queue=w287, element=w288, error in (no error)=w286) -> (error out=w285:errorcluster)  [unwired: 1 in, 2 out]
      }
      event "REFLECTEDTEMPERATURE": Value Change {
        n143 = event-data() -> ()  [unwired: 1 in, 1 out]
        n144 = Bundle("REFLECTEDTEMPERATURE"="REFLECTEDTEMPERATURE", Parameter."REFLECTEDTEMPERATURE") -> (w292:cluster{"REFLECTEDTEMPERATURE":sgl, T4})  [unwired: 1 in]
        n145 = To Variant(anything=w292) -> (Variant=w290:variant)
        n146 = Bundle By Name(cluster=cluster{"DATA":variant, "STATE":T2} {"DATA"=variant, "STATE"=enum."SETPARAMTER"} ("Element"), "DATA"=w290) -> (w298:cluster{"DATA":variant, "STATE":T2})
        n147 = Enqueue Element(queue=w296, element=w298, error in (no error)=w295) -> (error out=w294:errorcluster)  [unwired: 1 in, 2 out]
      }
      event "EMISSIVITY": Value Change {
        n148 = event-data() -> ()  [unwired: 1 in, 1 out]
        n149 = Bundle("EMISSIVITY"="EMISSIVITY", Parameter."EMISSIVITY") -> (w306:cluster{"EMISSIVITY":sgl, T4})  [unwired: 1 in]
        n150 = To Variant(anything=w306) -> (Variant=w305:variant)
        n151 = Bundle By Name(cluster=cluster{"DATA":variant, "STATE":T2} {"DATA"=variant, "STATE"=enum."SETPARAMTER"} ("Element"), "DATA"=w305) -> (w301:cluster{"DATA":variant, "STATE":T2})
        n152 = Enqueue Element(queue=w304, element=w301, error in (no error)=w303) -> (error out=w300:errorcluster)  [unwired: 1 in, 2 out]
      }
      event "SAVE - Button": Value Change {
        n153 = event-data() -> ()  [unwired: 1 in, 1 out]
        n154 = Enqueue Element(queue=w310, element=cluster{"DATA":variant, "STATE":T2} {"DATA"=variant, "STATE"=enum."SAVEIMAGE"} ("Element"), error in (no error)=w309) -> (error out=w308:errorcluster)  [unwired: 1 in, 2 out]
      }
      event "AMBIENTTEMPERATURE": Value Change {
        n155 = event-data() -> ()  [unwired: 1 in, 1 out]
        n156 = Bundle("AMBIENTTEMPERATURE"="AMBIENTTEMPERATURE", Parameter."AMBIENTTEMPERATURE") -> (w319:cluster{"AMBIENTTEMPERATURE":sgl, T4})  [unwired: 1 in]
        n157 = To Variant(anything=w319) -> (Variant=w315:variant)
        n158 = Bundle By Name(cluster=cluster{"DATA":variant, "STATE":T2} {"DATA"=variant, "STATE"=enum."SETPARAMTER"} ("Element"), "DATA"=w315) -> (w317:cluster{"DATA":variant, "STATE":T2})
        n159 = Enqueue Element(queue=w312, element=w317, error in (no error)=w313) -> (error out=w314:errorcluster)  [unwired: 1 in, 2 out]
      }
      event "HUMIDITY": Value Change {
        n160 = event-data() -> ()  [unwired: 1 in, 1 out]
        n161 = Bundle("HUMIDITY"="HUMIDITY", Parameter."HUMIDITY") -> (w328:cluster{"HUMIDITY":sgl, T4})  [unwired: 1 in]
        n162 = To Variant(anything=w328) -> (Variant=w324:variant)
        n163 = Bundle By Name(cluster=cluster{"DATA":variant, "STATE":T2} {"DATA"=variant, "STATE"=enum."SETPARAMTER"} ("Element"), "DATA"=w324) -> (w325:cluster{"DATA":variant, "STATE":T2})
        n164 = Enqueue Element(queue=w323, element=w325, error in (no error)=w322) -> (error out=w321:errorcluster)  [unwired: 1 in, 2 out]
      }
      event "EXIT - Button": Value Change {
        n165 = event-data() -> ()  [unwired: 1 in, 1 out]
        n166 = call "SubVI_CloseCamera.vi"("ErrorIn"=w331) -> ("ErrorOut"=w330:errorcluster)  [unwired: 9 in, 1 out]
        n167 = Enqueue Element(queue=w334, element=cluster{"DATA":variant, "STATE":T2} {"DATA"=variant, "STATE"=enum."EXIT"} ("Element"), error in (no error)=w330) -> (error out=w333:errorcluster)  [unwired: 1 in, 2 out]
      }
    }
    n168 = Unbundle By Name(w245) -> ("status"=w247:bool)
    n169 = Or(x=w247, y=w246) -> (x .or. y?=w248:bool)
  }
  n170 = Release Queue(queue=w10, error in (no error)=w9) -> ()  [unwired: 1 in, 3 out]
  n171 = Release Queue(queue=w8) -> ()  [unwired: 2 in, 3 out]
